vi "BRig_dataTrial_iReward.vi"() -> (2 "output_iReward":i32)   [LabVIEW 2014]
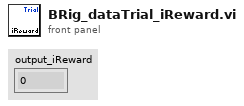
[diagram p1: front panel]
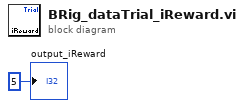
[diagram p0: block diagram]
diagram:
  "output_iReward" <- 5 ("output_iBlock")
